vi "GUI PJVS setup.vi"(10 "meas":T1={"Measurement ID"=enum."1 signal, 1 ADC, 1 PJVS", "Description"="3 phase, 3 ADC, 1 PJVS", "Switching matrix M"=[], "Signal frequency  (Hz)"=50.0, "Maximal signal amplitude (V)"=0.0, "PRs (samples)"=0, "PRe (samples)"=0, "MRs (s)"=0.0, "MRe (s)"=0.0, "Set PJVS frequency (Hz)"=50.0, "PJVS reference voltages (1 period, V)"=[], "Requiested PJVS steps"=10, "Sampling f (Hz)"=7000.0, "Trigger mode"=enum."Trigger every MX switch", "Timing matrix (periods)"=[], "Record length (multiples of M)"=1, "Calculated"={"Triggers to next path (line of sequence)"=[], "Record samples"=0, "Sample indexes of switches"=[], "PRs (s)"=0.0, "PRe (s)"=0.0, "MRs (samples)"=0, "MRe (samples)"=0, "Trigger frequency  (Hz)"=50.0, "Measurement druation (s)"=0.0, "Samples per step"=0.0, "QPMX Sequence"=[], "PJVS segments frequency (Hz)"=50.0}, "No of required digitizers"=0, "No of required transducers"=0, "Transducer correction files"=[], "Digitizer correction file"=path "", "Algorithm"="TWM-PWRFFT"} {"Calculated"."Trigger frequency  (Hz)" format="%#_6p"; "Record length (multiples of M)" min=1 step=1; "PJVS reference voltages (1 period, V)" format="%.9g"; "MRe (s)" format="%#_4p"; "MRs (s)" format="%#_4p"}, 11 "PJVS setup":T4={"PJVS type"=enum."AC-supraVOLTcontrol", "Status Refnum"=refnum, "AC-supraVOLTcontrol"={"IP address:port (0.0.0.0:0000)"="0.0.0.0:0000", "Timeouts"={"TCP Read & Write (ms)"=7000, "Sensors readout"=5000, "PJVS setup"=10000, "Nullmeter readout"=5000, "Multiplexer setup"=3000, "57XX setup"=15000, "Generator setup"=5000, "Synthesizer setup"=3000, "Sampler readout"=10000}, "Simulation mode"=FALSE, "Debug mode"=FALSE}, "NPL bias source"={"DataSocketCluster"={"Server Machine"="CZC", "Client Machine"="localhost", "Data"="P2", "TimeStamp"=0.0, "Count"=1, "Target Process"="General Server"}}, "Manual PJVS"={"PJVS frequency (Hz)"=0.0, "Reference voltages (V)"=[], "File with PJVS voltages"=path ""}, "VTT PJVS"={"some VTT only property"=""}} {"NPL bias source"."DataSocketCluster"."TimeStamp" format="%.2f"}) -> (2 "meas out":T1={"Measurement ID"=enum."1 signal, 1 ADC, 1 PJVS", "Description"="3 phase, 3 ADC, 1 PJVS", "Switching matrix M"=[], "Signal frequency  (Hz)"=50.0, "Maximal signal amplitude (V)"=0.0, "PRs (samples)"=0, "PRe (samples)"=0, "MRs (s)"=0.0, "MRe (s)"=0.0, "Set PJVS frequency (Hz)"=50.0, "PJVS reference voltages (1 period, V)"=[], "Requiested PJVS steps"=10, "Sampling f (Hz)"=7000.0, "Trigger mode"=enum."Trigger every MX switch", "Timing matrix (periods)"=[], "Record length (multiples of M)"=1, "Calculated"={"Triggers to next path (line of sequence)"=[], "Record samples"=0, "Sample indexes of switches"=[], "PRs (s)"=0.0, "PRe (s)"=0.0, "MRs (samples)"=0, "MRe (samples)"=0, "Trigger frequency  (Hz)"=50.0, "Measurement druation (s)"=0.0, "Samples per step"=0.0, "QPMX Sequence"=[], "PJVS segments frequency (Hz)"=50.0}, "No of required digitizers"=0, "No of required transducers"=0, "Transducer correction files"=[], "Digitizer correction file"=path "", "Algorithm"="TWM-PWRFFT"} {"Calculated"."Trigger frequency  (Hz)" format="%#_6p"; "Record length (multiples of M)" min=1 step=1; "PJVS reference voltages (1 period, V)" format="%.9g"; "MRe (s)" format="%#_4p"; "MRs (s)" format="%#_4p"}, 3 "PJVS setup out":T4={"PJVS type"=enum."AC-supraVOLTcontrol", "Status Refnum"=refnum, "AC-supraVOLTcontrol"={"IP address:port (0.0.0.0:0000)"="0.0.0.0:0000", "Timeouts"={"TCP Read & Write (ms)"=7000, "Sensors readout"=5000, "PJVS setup"=10000, "Nullmeter readout"=5000, "Multiplexer setup"=3000, "57XX setup"=15000, "Generator setup"=5000, "Synthesizer setup"=3000, "Sampler readout"=10000}, "Simulation mode"=FALSE, "Debug mode"=FALSE}, "NPL bias source"={"DataSocketCluster"={"Server Machine"="CZC", "Client Machine"="localhost", "Data"="P2", "TimeStamp"=0.0, "Count"=1, "Target Process"="General Server"}}, "Manual PJVS"={"PJVS frequency (Hz)"=0.0, "Reference voltages (V)"=[], "File with PJVS voltages"=path ""}, "VTT PJVS"={"some VTT only property"=""}} {"NPL bias source"."DataSocketCluster"."TimeStamp" format="%.2f"})   [LabVIEW 2020]
doc: "Use this template to build a producer/consumer design pattern with events to produce queue items. Use this design pattern instead of the User Interface Event Handler pattern for user interfaces when you want to execute code asynchronously in response to an event without slowing the user interface responsiveness."
uses:
  General PJVS driver/Type definitions/PJVS Setup.ctl
  General PJVS driver/Type definitions/PJVS Type.ctl
  PJVS drivers/acsvcontrol-driver/build/ACSVcontrol-driver_0.2.1.0.llb/Timeouts.ctl
  PJVS drivers/JV modified NPL Bias source/DataSocketCluster external.ctl
  Measurement/Type definitions/Measuement properties.ctl
  Measurement/Type definitions/Measurement ID.ctl
  Measurement/Type definitions/Trigger mode.ctl
  <vilib>/Utility/error.llb/Error Cluster From Error Code.vi
  <vilib>/Utility/file.llb/Read Delimited Spreadsheet (DBL).vi
  <vilib>/ErrorRing/Error Ring.xnode
  external libraries/varilib/varilib.lvlib
  PJVS drivers/acsvcontrol-driver/build/ACSVcontrol-driver_0.2.1.0.llb/ACSVcontrol-driver.lvlib
panel:
  out "gui_elements":refnum<vi>[](array[refnum])
  out "Status":string
  out "error out":errorcluster
  in  "save_and_quit":bool
  in  "PJVS type tab":T8(tab)
  in  "Debug mode":bool
  in  "IP address:port (0.0.0.0:0000)":string
  in  "Timeouts":T6={"TCP Read & Write (ms)"=7000, "Sensors readout"=5000, "PJVS setup"=5000, "Nullmeter readout"=5000, "Multiplexer setup"=3000, "57XX setup"=15000, "Generator setup"=5000, "Synthesizer setup"=3000, "Sampler readout"=10000}
  in  "Simulation mode":bool
  out "DataSocketCluster":T7 {"TimeStamp" format="%.2f"}
  out "manual: no of voltages":i32 caption="Number of reference voltages in the table"
  in  "File with PJVS voltages":path caption="File with reference voltages"
  in  "load voltages":bool
  in  "manual: reference voltages (V)":dbl[](array[numeric]) caption="Reference voltages (V)\n(voltages of PJVS steps)" format="%0.12g"
  in  "Set PJVS frequency (Hz)":dbl caption="PJVS frequency (Hz)\n(frequency of one PJVS period)" format="%#_9g"
  in  "test":bool
  in  "cancel":bool
  # "For a dummy PJVS, set \"AC-supraVOLTcontrol\" and set \"Simulation mode\". In this way this software\ncan be tested without running real PJVS."
  # "Manual mode help\nEither enter reference voltages manually into the table, or select a file and load it using the button. The file must be a text file with PJVS values in a first collumn of a tab or comma separated table.\n\nDo not forget to set PJVS frequency."
  # "#VTT add something here"
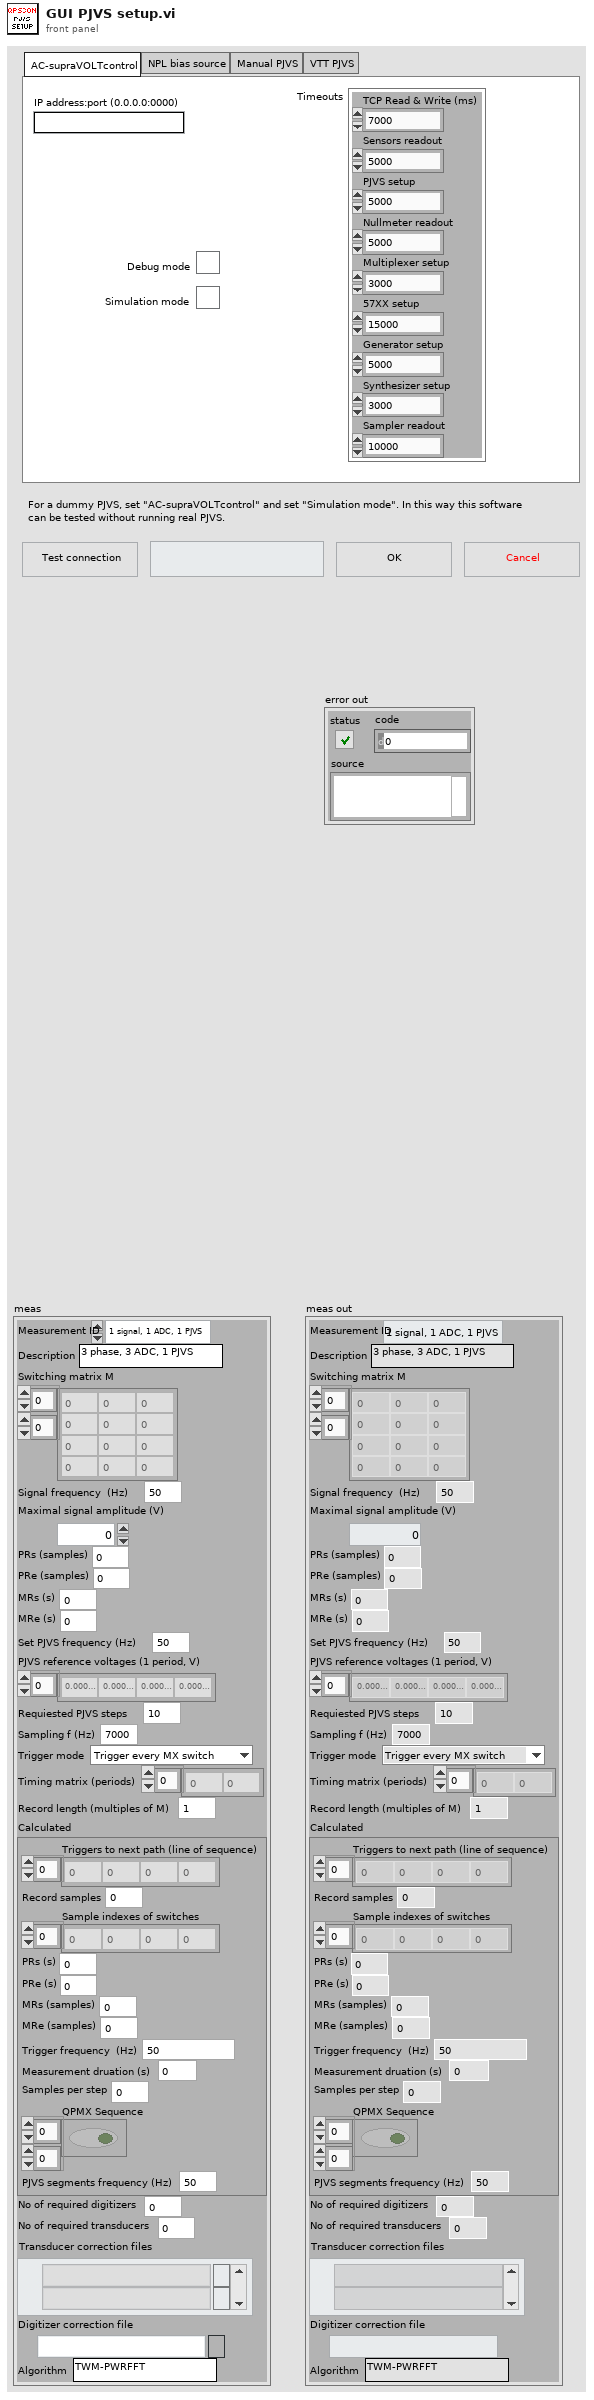
[diagram p1: front panel]
types:
  T1 = typedef "Measuement properties.ctl" = cluster{"Measurement ID":T2, "Description":string, "Switching matrix M":i32[][], "Signal frequency  (Hz)":dbl, "Maximal signal amplitude (V)":dbl, "PRs (samples)":u32, "PRe (samples)":u32, "MRs (s)":dbl, "MRe (s)":dbl, "Set PJVS frequency (Hz)":dbl, "PJVS reference voltages (1 period, V)":dbl[], "Requiested PJVS steps":u32, "Sampling f (Hz)":dbl, "Trigger mode":T3, "Timing matrix (periods)":i32[], "Record length (multiples of M)":u32, "Calculated":cluster{"Triggers to next path (line of sequence)":u32[], "Record samples":u32, "Sample indexes of switches":u32[], "PRs (s)":dbl, "PRe (s)":dbl, "MRs (samples)":i32, "MRe (samples)":i32, "Trigger frequency  (Hz)":dbl, "Measurement druation (s)":dbl, "Samples per step":dbl, "QPMX Sequence":bool[][], "PJVS segments frequency (Hz)":dbl}, "No of required digitizers":u32, "No of required transducers":u32, "Transducer correction files":path[], "Digitizer correction file":path, "Algorithm":string}
  T2 = typedef "Measurement ID.ctl" = enum16{"Manual setup", "1 signal, 1 ADC, 1 PJVS", "1 phase (U, I), 1 ADC, 1 PJVS", "1 phase (U, I), 2 ADC, 1 PJVS", "1 phase (U, I), 3 ADC, 1 PJVS", "3 phases (U1..3, I1..3), 3 ADC, 1 PJVS"}
  T3 = typedef "Trigger mode.ctl" = enum16{"Trigger every MX switch", "Trigger every sample"}
  T4 = typedef "PJVS Setup.ctl" = cluster{"PJVS type":T5, "Status Refnum":refnum<vi>, "AC-supraVOLTcontrol":cluster{"IP address:port (0.0.0.0:0000)":string, "Timeouts":T6, "Simulation mode":bool, "Debug mode":bool}, "NPL bias source":cluster{"DataSocketCluster":T7}, "Manual PJVS":cluster{"PJVS frequency (Hz)":dbl, "Reference voltages (V)":dbl[], "File with PJVS voltages":path}, "VTT PJVS":cluster{"some VTT only property":string}}
  T5 = typedef "PJVS Type.ctl" = enum16{"AC-supraVOLTcontrol", "JV modified NPL bias control", "Manual PJVS", "VTT PJVS"}
  T6 = typedef "ACSVcontrol-driver.lvlib/Timeouts.ctl" = cluster{"TCP Read & Write (ms)":i32, "Sensors readout":i32, "PJVS setup":i32, "Nullmeter readout":i32, "Multiplexer setup":i32, "57XX setup":i32, "Generator setup":i32, "Synthesizer setup":i32, "Sampler readout":i32}
  T7 = typedef "DataSocketCluster external.ctl" = cluster{"Server Machine":string, "Client Machine":string, "Data":string, "TimeStamp":dbl, "Count":i32, "Target Process":string}
  T8 = enum32{"AC-supraVOLTcontrol", "NPL bias source", "Manual PJVS", "VTT PJVS"}
  T9 = cluster{"IP address:port (0.0.0.0:0000)":string, "Timeouts":T6, "Simulation mode":bool, "Debug mode":bool}
  T10 = cluster{"PJVS frequency (Hz)":dbl, "Reference voltages (V)":dbl[], "File with PJVS voltages":path}
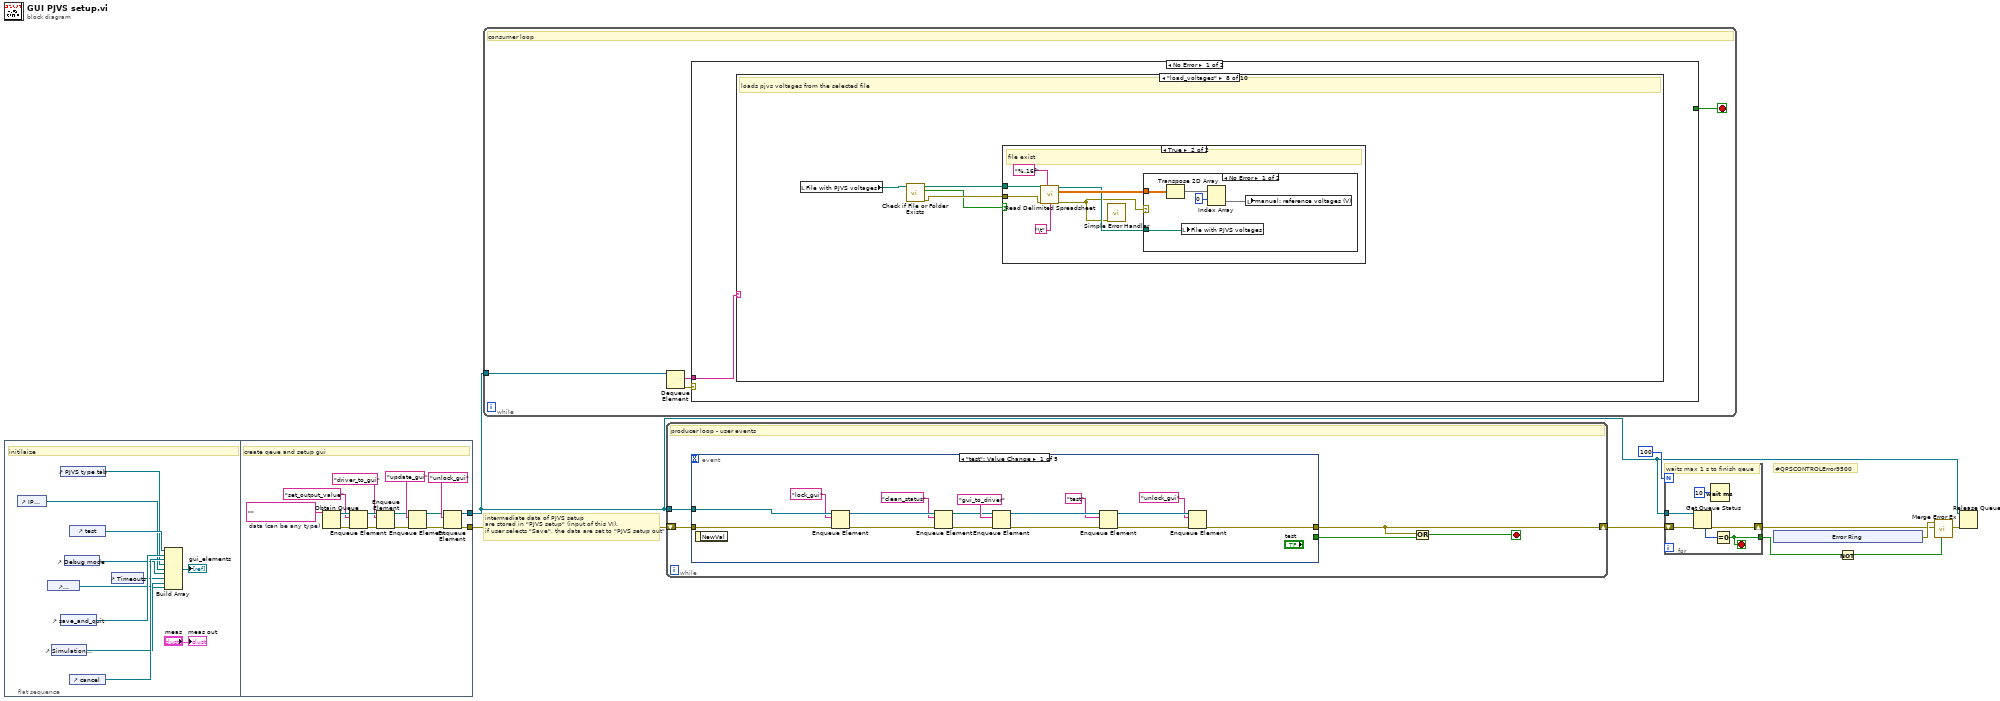
[diagram p0: block diagram]
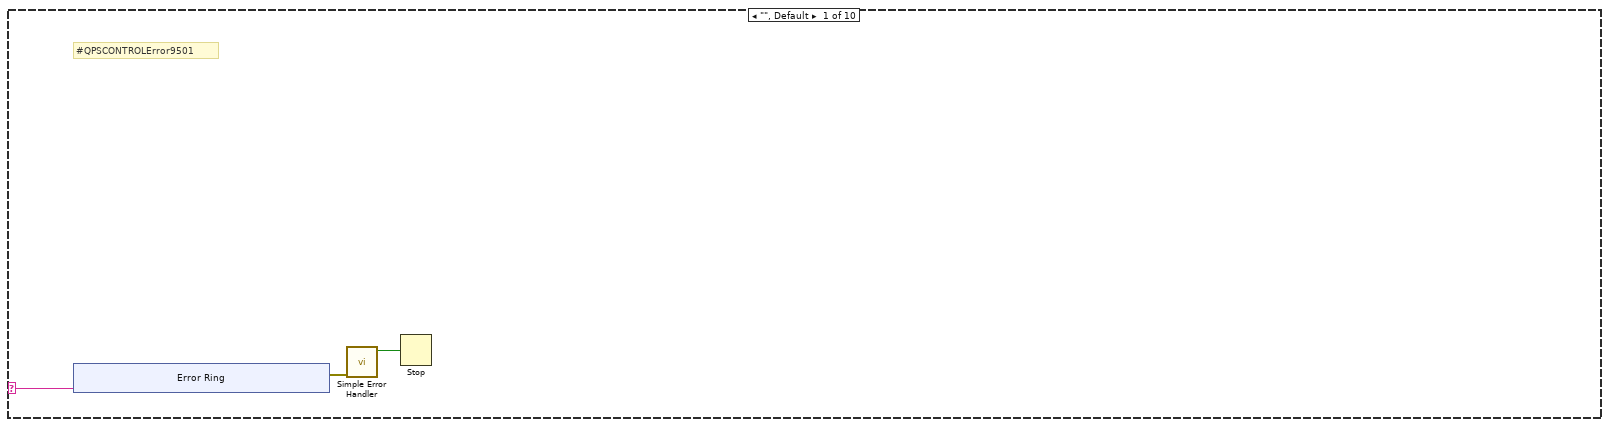
[diagram p2: hidden frame]
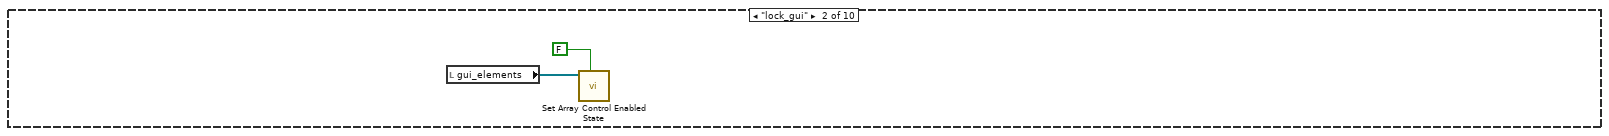
[diagram p3: hidden frame]
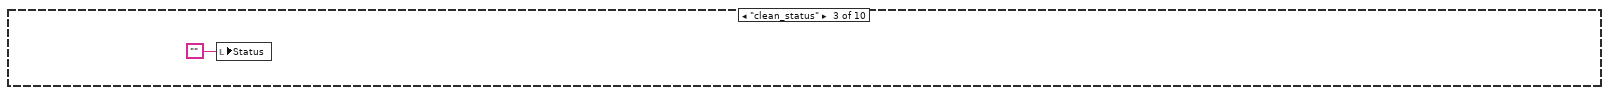
[diagram p4: hidden frame]
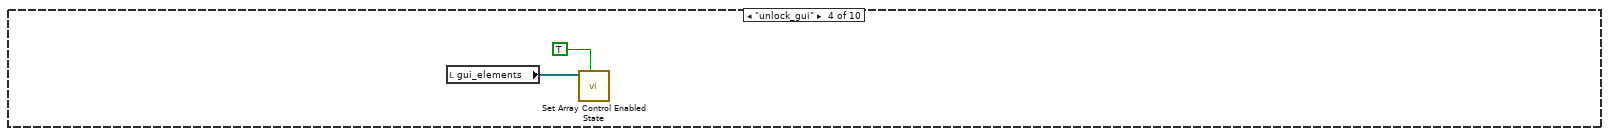
[diagram p5: hidden frame]
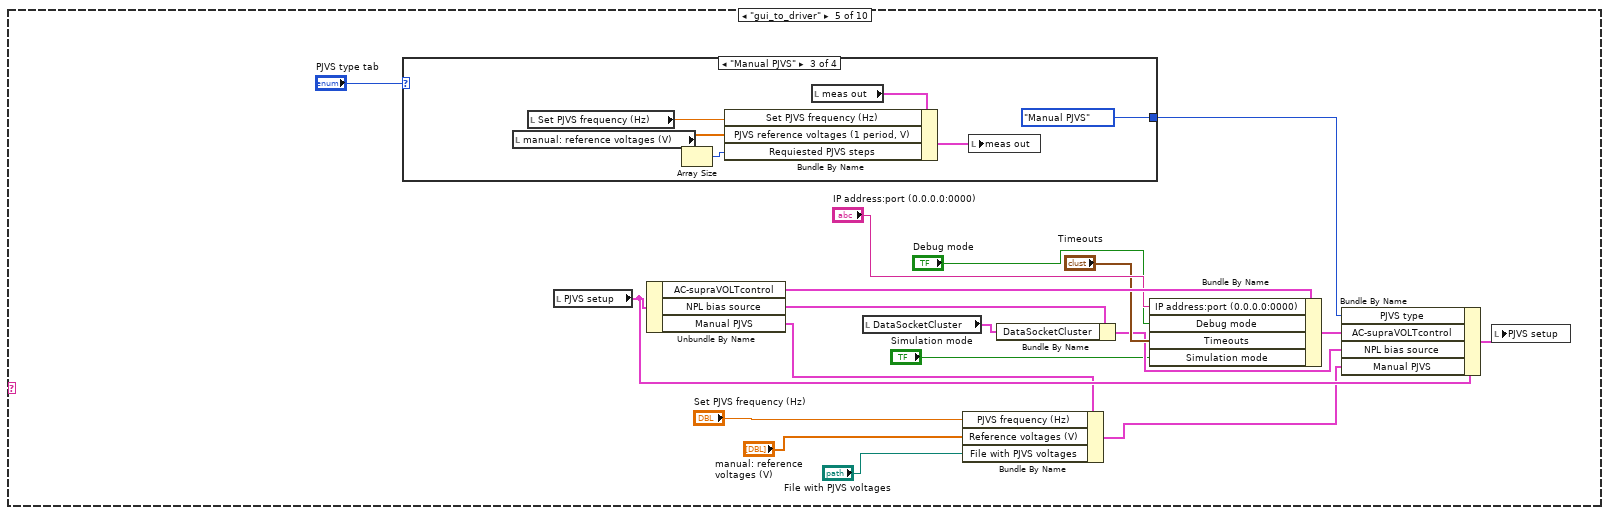
[diagram p6: hidden frame]
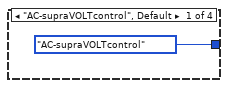
[diagram p7: hidden frame]
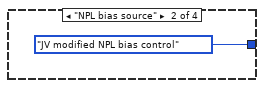
[diagram p8: hidden frame]
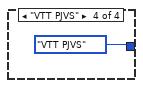
[diagram p9: hidden frame]
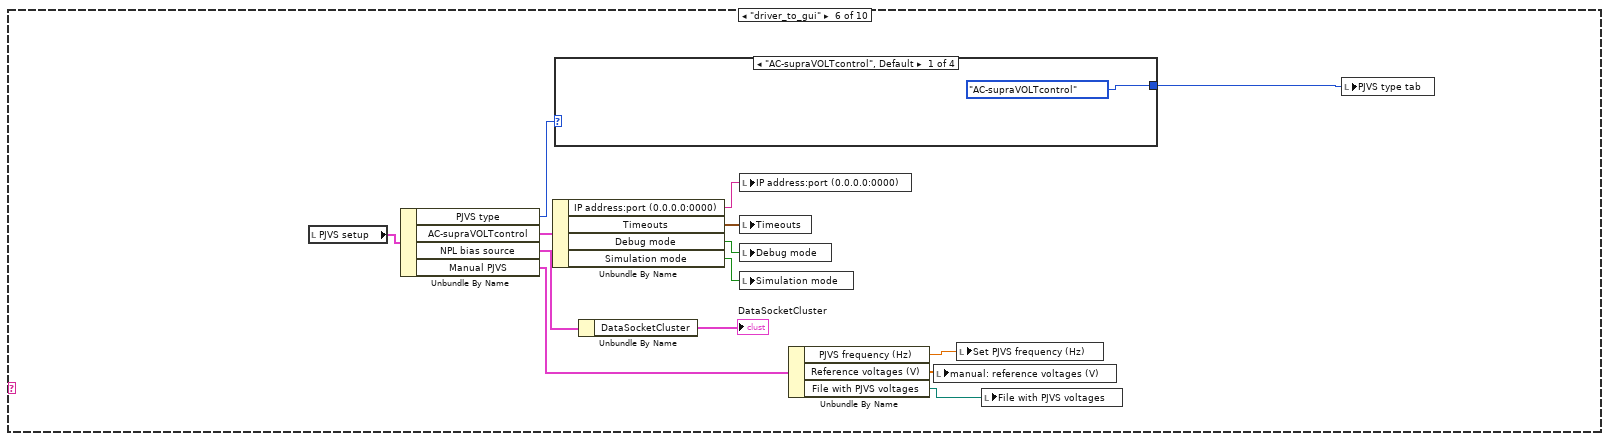
[diagram p10: hidden frame]
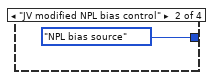
[diagram p11: hidden frame]
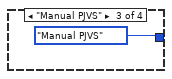
[diagram p12: hidden frame]
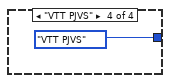
[diagram p13: hidden frame]
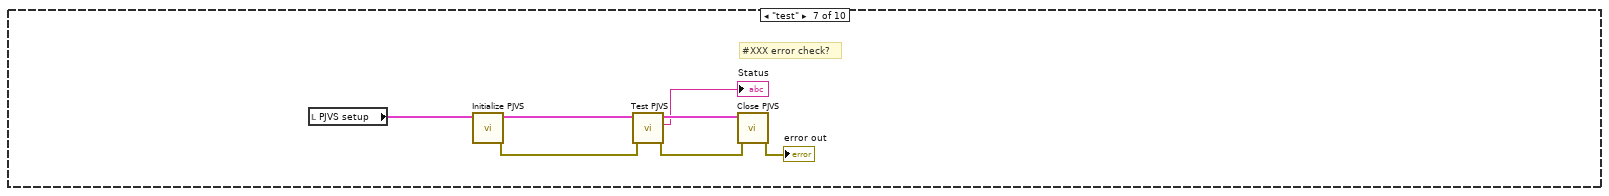
[diagram p14: hidden frame]
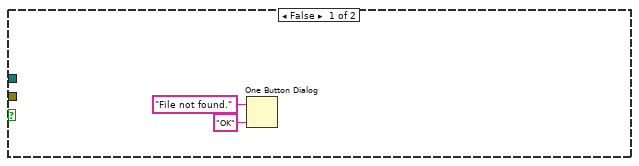
[diagram p15: hidden frame]
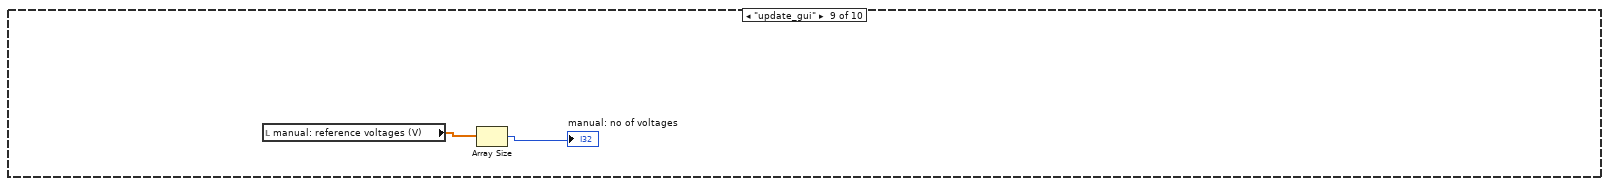
[diagram p17: hidden frame]
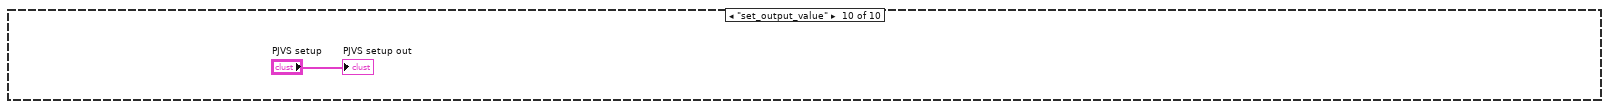
[diagram p18: hidden frame]
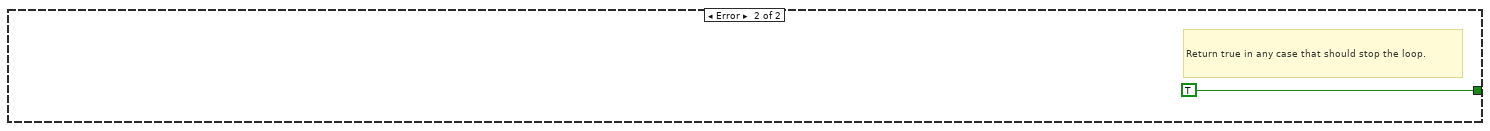
[diagram p19: hidden frame]
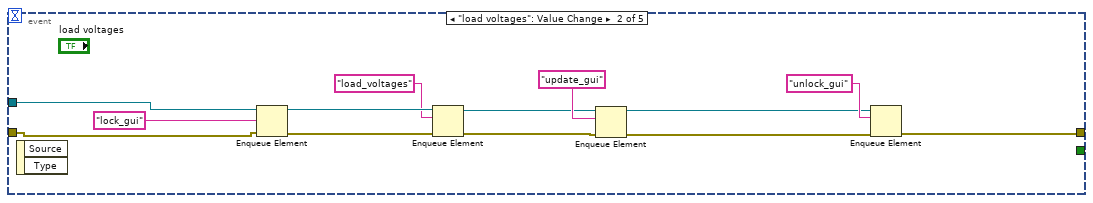
[diagram p20: hidden frame]
diagram:
  # "#QPSCONTROLError9500"
  # "intermediate data of PJVS setup\nare stored in \"PJVS setup\" (input of this VI),\nif user selects \"Save\", the data are set to \"PJVS setup out\""
  n1 = flat-sequence {
    tunnel: [w28] -> w2
    tunnel: [w26] -> w1
    frame #0 {
      # "initilaize"
      n2 = control-ref of="IP address:port (0.0.0.0:0000)"() -> (w16:refnum<vi>)
      n3 = control-ref of="DataSocketCluster"() -> (w11:refnum<vi>)
      n4 = control-ref of="Simulation mode"() -> (w13:refnum<vi>)
      n5 = control-ref of="PJVS type tab"() -> (w17:refnum<vi>)
      n6 = control-ref of="save_and_quit"() -> (w19:refnum<vi>)
      n7 = control-ref of="Debug mode"() -> (w12:refnum<vi>)
      n8 = control-ref of="test"() -> (w20:refnum<vi>)
      n9 = control-ref of="cancel"() -> (w18:refnum<vi>)
      n10 = control-ref of="Timeouts"() -> (w15:refnum<vi>)
      n11 = Build Array(w20, w19, w18, w17, w16, w12, w15, w11, w13) -> (→"gui_elements":refnum<vi>[])
      "meas out" <- "meas"
    }
    frame #1 {
      w27 = ""  # data (can be any type)
      # "create qeue and setup gui"
      n12 = Obtain Queue(element data type=w27) -> (queue out=w32:refnum<queue>, error out=w34:errorcluster)  [unwired: 4 in, 1 out]
      n13 = Enqueue Element(queue=w32, element="set_output_value", error in (no error)=w34) -> (queue out=w33:refnum<queue>, error out=w35:errorcluster)  [unwired: 1 in, 1 out]
      n14 = Enqueue Element(queue=w33, element="driver_to_gui", error in (no error)=w35) -> (queue out=w24:refnum<queue>, error out=w21:errorcluster)  [unwired: 1 in, 1 out]
      n15 = Enqueue Element(queue=w24, element="update_gui", error in (no error)=w21) -> (queue out=w23:refnum<queue>, error out=w22:errorcluster)  [unwired: 1 in, 1 out]
      n16 = Enqueue Element(queue=w23, element="unlock_gui", error in (no error)=w22) -> (queue out=w28:refnum<queue>, error out=w26:errorcluster)  [unwired: 1 in, 1 out]
    }
  }
  n17 = while {
    tunnel: w2 -> [w39]
    stop <- w36 stop-if-true
    # "consumer loop"
    n18 = Dequeue Element(queue=w39) -> (element=w37:string, error out=w38:errorcluster)  [unwired: 2 in, 2 out]
    n19 = case shown="No Error" w38 {
      tunnel: w37 -> [w40 _]
      tunnel: [_ TRUE] -> w36
      frame No Error {
        n20 = case shown="\"load_voltages\"" w40 {
          selector: w40 -> [w41 _ _ _ _ _ _ _ _ _]
          frame "", Default {
            # "#QPSCONTROLError9501"
            n21 = xnode "Error Ring"("parameter 0"=w41) -> ("error out"=w43:errorcluster)
            n22 = call <vilib>:"Simple Error Handler.vi"("error in (no error)"=w43) -> ("error?"=w42:bool)  [unwired: 4 in, 4 out]
            n23 = Stop(stop? (T)=w42) -> ()
          }
          frame "lock_gui" {
            n24 = local read "gui_elements"() -> (w52:refnum<vi>[])
            n25 = call "Set Array Control Enabled State.vi"("enabled (T)"=FALSE, "reference array in"=w52) -> ()  [unwired: 8 in, 2 out]
          }
          frame "clean_status" {
            n26 = local write "Status"("") -> ()
          }
          frame "unlock_gui" {
            n27 = local read "gui_elements"() -> (w55:refnum<vi>[])
            n28 = call "Set Array Control Enabled State.vi"("enabled (T)"=TRUE, "reference array in"=w55) -> ()  [unwired: 8 in, 2 out]
          }
          frame "gui_to_driver" {
            n29 = case shown="\"Manual PJVS\"" "PJVS type tab" {
              tunnel: [PJVS_Type."AC-supraVOLTcontrol" ("PJVS type") PJVS_Type."JV modified NPL bias control" ("PJVS type") PJVS_Type."Manual PJVS" ("PJVS type") PJVS_Type."VTT PJVS" ("PJVS type")] -> w71
              frame "AC-supraVOLTcontrol", Default {
              }
              frame "NPL bias source" {
              }
              frame "Manual PJVS" {
                n30 = local read "manual: reference voltages (V)"() -> (w77:dbl[])
                n31 = local read "Set PJVS frequency (Hz)"() -> (w78:dbl)
                n32 = Array Size(array=w77) -> (size(s)=w76:i32)
                n33 = local read "meas out"() -> (w80:T1)
                n34 = Bundle By Name(cluster=w80, "Set PJVS frequency (Hz)"=w78, "PJVS reference voltages (1 period, V)"=w77, "Requiested PJVS steps"=w76) -> (w79:T1)
                n35 = local write "meas out"(w79) -> ()
              }
              frame "VTT PJVS" {
              }
            }
            n36 = local read "PJVS setup"() -> (w66:T4)
            n37 = Unbundle By Name(w66) -> ("AC-supraVOLTcontrol"=w70:T9, "NPL bias source"=w65:cluster{"DataSocketCluster":T7}, "Manual PJVS"=w60:T10)
            n38 = local read "DataSocketCluster"() -> (w61:T7)
            n39 = Bundle By Name(cluster=w60, "PJVS frequency (Hz)"="Set PJVS frequency (Hz)", "Reference voltages (V)"="manual: reference voltages (V)", "File with PJVS voltages"="File with PJVS voltages") -> (w59:T10)
            n40 = Bundle By Name(cluster=w65, "DataSocketCluster"=w61) -> (w64:cluster{"DataSocketCluster":T7})
            n41 = Bundle By Name(cluster=w70, "IP address:port (0.0.0.0:0000)"="IP address:port (0.0.0.0:0000)", "Debug mode"="Debug mode", "Timeouts"="Timeouts", "Simulation mode"="Simulation mode") -> (w69:T9)
            n42 = Bundle By Name(cluster=w66, "PJVS type"=w71, "AC-supraVOLTcontrol"=w69, "NPL bias source"=w64, "Manual PJVS"=w59) -> (w73:T4)
            n43 = local write "PJVS setup"(w73) -> ()
          }
          frame "driver_to_gui" {
            n44 = local read "PJVS setup"() -> (w87:T4)
            n45 = Unbundle By Name(w87) -> ("PJVS type"=w96:T5, "AC-supraVOLTcontrol"=w95:T9, "NPL bias source"=w92:cluster{"DataSocketCluster":T7}, "Manual PJVS"=w86:T10)
            n46 = Unbundle By Name(w95) -> ("IP address:port (0.0.0.0:0000)"=w94:string, "Timeouts"=w93:T6, "Debug mode"=w90:bool, "Simulation mode"=w91:bool)
            n47 = case shown="\"AC-supraVOLTcontrol\", Default" w96 {
              tunnel: [T8."AC-supraVOLTcontrol" ("PJVS type tab") T8."NPL bias source" ("PJVS type tab") T8."Manual PJVS" ("PJVS type tab") T8."VTT PJVS" ("PJVS type tab")] -> w88
              frame "AC-supraVOLTcontrol", Default {
              }
              frame "JV modified NPL bias control" {
              }
              frame "Manual PJVS" {
              }
              frame "VTT PJVS" {
              }
            }
            n48 = Unbundle By Name(w92) -> ("DataSocketCluster"=→"DataSocketCluster":T7)
            n49 = local write "IP address:port (0.0.0.0:0000)"(w94) -> ()
            n50 = local write "Timeouts"(w93) -> ()
            n51 = local write "Debug mode"(w90) -> ()
            n52 = local write "Simulation mode"(w91) -> ()
            n53 = Unbundle By Name(w86) -> ("PJVS frequency (Hz)"=w84:dbl, "Reference voltages (V)"=w85:dbl[], "File with PJVS voltages"=w83:path)
            n54 = local write "manual: reference voltages (V)"(w85) -> ()
            n55 = local write "Set PJVS frequency (Hz)"(w84) -> ()
            n56 = local write "File with PJVS voltages"(w83) -> ()
            n57 = local write "PJVS type tab"(w88) -> ()
          }
          frame "test" {
            # "#XXX error check?"
            n58 = local read "PJVS setup"() -> (w103:T4)
            n59 = call "Initialize PJVS.vi"("PJVS setup"=w103) -> ("error out"=w107:errorcluster, "PJVS setup out"=w104:T4)  [unwired: 9 in]
            n60 = call "Test PJVS.vi"("error in (pass through)"=w107, "PJVS setup"=w104) -> ("error out"=w106:errorcluster, "Status"=→"Status":string, "PJVS setup out"=w105:T4)  [unwired: 7 in]
            n61 = call "Close PJVS.vi"("error in (pass through)"=w106, "PJVS setup"=w105) -> ("error out"=→"error out":errorcluster)  [unwired: 8 in, 1 out]
          }
          frame "load_voltages" {
            # "loads pjvs voltages from the selected file"
            n62 = local read "File with PJVS voltages"() -> (w111:path)
            n63 = call <vilib>:"Check if File or Folder Exists.vi"("path"=w111) -> ("error out"=w109:errorcluster, "file or folder exists?"=w108:bool, "dup path"=w110:path)  [unwired: 8 in]
            n64 = case shown="True" w108 {
              tunnel: w110 -> [_ w117]
              tunnel: w109 -> [_ w116]
              frame False {
                n65 = One Button Dialog(message="File not found.", button name ("OK")="OK") -> ()  [unwired: 1 out]
              }
              frame True {
                # "file exist"
                n66 = call-poly <vilib>:"Read Delimited Spreadsheet.vi"("file path (dialog if empty)"=w117, "format (%.3f)"="%.16f", "error in (no error)"=w116, "delimiter (\\t)"="\t") -> ("new file path (Not A Path if cancelled)"=w115:path, "all rows"=w118:dbl[][], "error out"=w114:errorcluster)  [unwired: 6 in, 3 out]
                n67 = call <vilib>:"Simple Error Handler.vi"("error in (no error)"=w114) -> ()  [unwired: 4 in, 5 out]
                n68 = case shown="No Error" w114 {
                  tunnel: w118 -> [w123 _]
                  tunnel: w115 -> [w121 _]
                  frame No Error {
                    n69 = Transpose 2D Array(2D array=w123) -> (transposed array=w122:dbl[][])
                    n70 = local write "File with PJVS voltages"(w121) -> ()
                    n71 = Index Array(array=w122, index (row)=0 ("index")) -> (element=w124:dbl[])  [unwired: 1 in]
                    n72 = local write "manual: reference voltages (V)"(w124) -> ()
                  }
                  frame Error {
                  }
                }
              }
            }
          }
          frame "update_gui" {
            n73 = local read "manual: reference voltages (V)"() -> (w127:dbl[])
            n74 = Array Size(array=w127) -> (size(s)=→"manual: no of voltages":i32)
          }
          frame "set_output_value" {
            "PJVS setup out" <- "PJVS setup"
          }
        }
      }
      frame Error {
        # "Return true in any case that should stop the loop."
      }
    }
  }
  n75 = while {
    shift-right: [w130] -> w5
    shift-left: w1 -> [w133]
    tunnel: w2 -> [w134]
    stop <- w131 stop-if-true
    # "producer loop - user events"
    n76 = event shown="[0] \"test\": Value Change" {
      selector: _ -> [_ _ _ _ _]
      dyn-events: _ -> [_ _ _ _ _]
      timeout: _ -> [_ _ _ _ _]
      tunnel: w134 -> [w141 w157 w165 w172 _]
      tunnel: w133 -> [w142 w158 w166 w169 w177]
      tunnel: [w145 w156 w164 w168 w177] -> w130
      tunnel: [_ _ _ TRUE ("cancel") TRUE ("cancel")] -> w132
      event "test": Value Change {
        n77 = event-data() -> ()  [unwired: 1 in, 1 out]
        n78 = Enqueue Element(queue=w141, element="lock_gui", error in (no error)=w142) -> (queue out=w138:refnum<queue>, error out=w139:errorcluster)  [unwired: 1 in, 1 out]
        n79 = Enqueue Element(queue=w138, element="clean_status", error in (no error)=w139) -> (queue out=w136:refnum<queue>, error out=w137:errorcluster)  [unwired: 1 in, 1 out]
        n80 = Enqueue Element(queue=w136, element="gui_to_driver", error in (no error)=w137) -> (queue out=w148:refnum<queue>, error out=w149:errorcluster)  [unwired: 1 in, 1 out]
        n81 = Enqueue Element(queue=w148, element="test", error in (no error)=w149) -> (queue out=w144:refnum<queue>, error out=w146:errorcluster)  [unwired: 1 in, 1 out]
        n82 = Enqueue Element(queue=w144, element="unlock_gui", error in (no error)=w146) -> (error out=w145:errorcluster)  [unwired: 1 in, 2 out]
      }
      event "load voltages": Value Change {
        n83 = event-data() -> ()  [unwired: 1 in, 2 out]
        n84 = Enqueue Element(queue=w157, element="lock_gui", error in (no error)=w158) -> (queue out=w162:refnum<queue>, error out=w163:errorcluster)  [unwired: 1 in, 1 out]
        n85 = Enqueue Element(queue=w162, element="load_voltages", error in (no error)=w163) -> (queue out=w153:refnum<queue>, error out=w154:errorcluster)  [unwired: 1 in, 1 out]
        n86 = Enqueue Element(queue=w153, element="update_gui", error in (no error)=w154) -> (queue out=w152:refnum<queue>, error out=w151:errorcluster)  [unwired: 1 in, 1 out]
        n87 = Enqueue Element(queue=w152, element="unlock_gui", error in (no error)=w151) -> (error out=w156:errorcluster)  [unwired: 1 in, 2 out]
      }
      event "manual: reference voltages (V)": Value Change {
        n88 = event-data() -> ()  [unwired: 1 in, 2 out]
        n89 = Enqueue Element(queue=w165, element="update_gui", error in (no error)=w166) -> (error out=w164:errorcluster)  [unwired: 1 in, 2 out]
      }
      event "save_and_quit": Value Change {
        n90 = event-data() -> ()  [unwired: 1 in, 1 out]
        n91 = Enqueue Element(queue=w172, element="gui_to_driver", error in (no error)=w169) -> (queue out=w171:refnum<queue>, error out=w170:errorcluster)  [unwired: 1 in, 1 out]
        n92 = Enqueue Element(queue=w171, element="set_output_value", error in (no error)=w170) -> (error out=w168:errorcluster)  [unwired: 1 in, 2 out]
      }
      event "cancel": Value Change; Panel Close {
        n93 = event-data() -> ()  [unwired: 1 in, 2 out]
      }
    }
    n94 = Or(x=w130, y=w132) -> (x .or. y?=w131:bool)
  }
  n95 = for {
    N: 100 -> [_]
    tunnel: w2 -> [w183]
    shift-right: [w181] -> w6
    shift-left: w5 -> [w182]
    tunnel: [w178] -> w3
    stop <- w178 stop-if-true
    # "waits max 1 s to finish qeue"
    n96 = Get Queue Status(queue=w183, error in (no error)=w182) -> (error out=w181:errorcluster, # elements in queue=w179:i32)  [unwired: 1 in, 6 out]
    n97 = Wait (ms)(milliseconds to wait=u32 10) -> ()  [unwired: 1 out]
    n98 = Equal To 0?(x=w179) -> (x = 0?=w178:bool)
  }
  n99 = xnode "Error Ring"() -> ("error out"=w7:errorcluster)
  n100 = Not(x=w3) -> (.not. x?=w8:bool)
  n101 = call "Merge Error Ex.vi"("Is error? (False)"=w8, "main error in (no error)"=w6, "second error in"=w7) -> ("error out"=w4:errorcluster)  [unwired: 8 in]
  n102 = Release Queue(queue=w2, error in (no error)=w4) -> ()  [unwired: 1 in, 3 out]
